vi "NewRoom.vi"(8 "error in (no error)":errorcluster, 11 "RoomNumber":i32) -> (0 "error out":errorcluster, 3 "Room":refnum<class "Room.lvclass">)   [LabVIEW 2020, in "Room.lvclass"]
uses:
  Room.lvclass
  Room.lvclass/Room.ctl
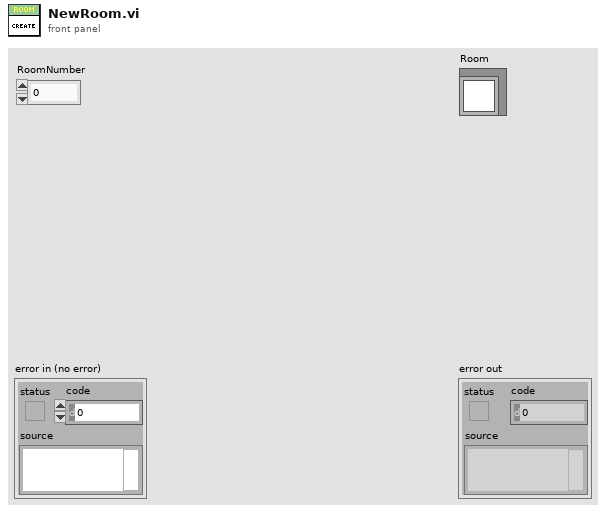
[diagram p1: front panel]
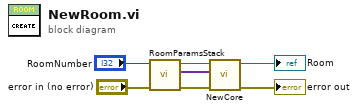
[diagram p0: block diagram]
diagram:
  n1 = call "RoomParamsStack.vi"("error in (no error)"="error in (no error)", "RoomNumber"="RoomNumber") -> ("error out"=w7:errorcluster, "HierarchyParams"=w6:variant[], "Room"=w5:refnum<class "Room.lvclass">)  [unwired: 7 in]
  n2 = call-dynamic "NewCore.vi"("error in (no error)"=w7, "ParamsArray"=w6, "Room"=w5) -> ("error out"=→"error out":errorcluster, "Room"=→"Room":refnum<class "Room.lvclass">)  [unwired: 7 in]
